vi "Temperature Monitor.vi"() -> ()   [LabVIEW 2017]
doc: "This VI is the solution to an exercise in the LabVIEW Core 1 course.\n\nIt uses a While Loop and shift registers to average data. No hardware is necessary."
panel:
  in  "Stop Button":bool
  out "Temperature History":cluster{dbl, "Temperature Value":dbl}(graph)
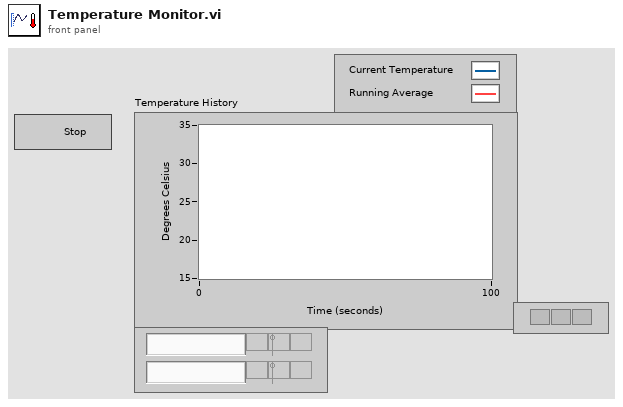
[diagram p1: front panel]
types:
  T1 = enum16{"open", "replace", "create", "open or create", "replace or create", "replace or create with confirmation"}
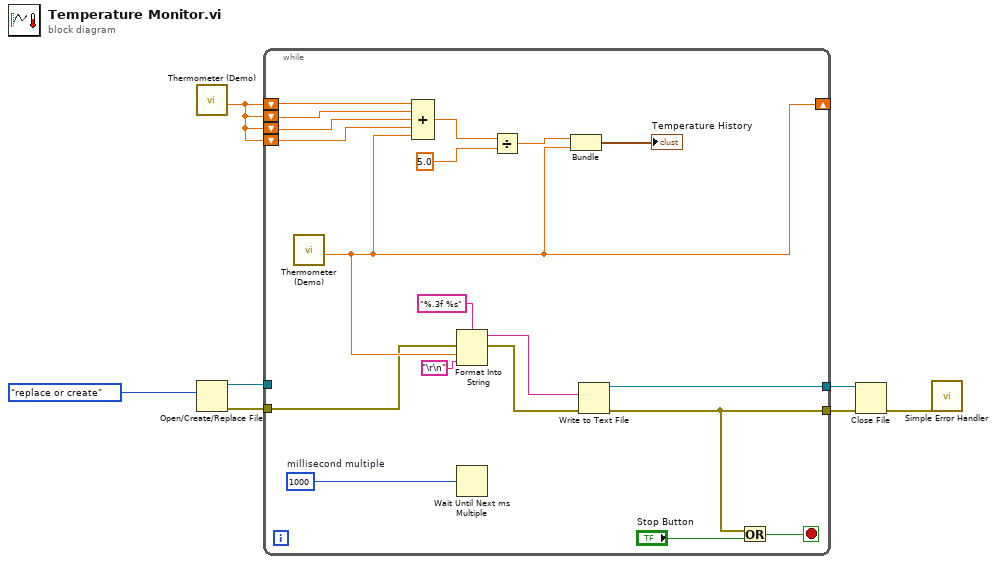
[diagram p0: block diagram]
diagram:
  n1 = call "Thermometer (Demo).vi"() -> ("Temperature Value"=w7:dbl)  [unwired: 11 in]
  n2 = Open/Create/Replace File(operation (0:open)=T1."replace or create") -> (refnum out=w3:refnum<file>, error out=w2:errorcluster)  [unwired: 5 in, 1 out]
  n3 = while {
    shift-right: [w17] -> _
    shift-left: w7 -> [w23]
    shift-left: w7 -> [w22]
    shift-left: w7 -> [w21]
    shift-left: w7 -> [w20]
    tunnel: [w10] -> w6
    tunnel: [w13] -> w5
    tunnel: w3 -> [_]
    tunnel: w2 -> [w8]
    stop <- w11 stop-if-true
    w26 = u32 1000  # millisecond multiple
    n4 = call "Thermometer (Demo).vi"() -> ("Temperature Value"=w17:dbl)  [unwired: 11 in]
    n5 = Compound Arithmetic op=ADD(w23, w22, w21, w20, w17) -> (w25:dbl)
    n6 = Format Into String(format string="%.3f %s", error in=w8, w17, "\r\n") -> (resulting string=w14:string, error out=w15:errorcluster)  [unwired: 1 in]
    n7 = Wait Until Next ms Multiple(millisecond multiple=w26) -> ()  [unwired: 1 out]
    n8 = Divide(x=w25, y=5.0 ("x/y")) -> (x/y=w18:dbl)
    n9 = Bundle(w18, "Temperature Value"=w17) -> (→"Temperature History":cluster{dbl, "Temperature Value":dbl})  [unwired: 1 in]
    n10 = Write to Text File(text=w14, error in=w15) -> (refnum out=w13:refnum<file>, error out=w10:errorcluster)  [unwired: 2 in, 1 out]
    n11 = Or(x=w10, y="Stop Button") -> (x .or. y?=w11:bool)
  }
  n12 = Close File(refnum=w5, error in=w6) -> (error out=w4:errorcluster)  [unwired: 1 out]
  n13 = call <vilib>:"Simple Error Handler.vi"("error in (no error)"=w4) -> ()  [unwired: 4 in, 5 out]
